vi "PH_DIM.get Boolean Status.vi"(2 "no link":bool, 3 "typeDescriptor":string, 4 "data":i8[](array[numeric]), 5 "quality":i32) -> (0 "further information":string, 1 "Status":T1 items=["no info", "off/false/out", "on/true/in", "Failure", "Alarm", "Status 1", "Status 2", "Status 3"])   [LabVIEW 2014, in "PH_Common.lvlib"]
doc: "This VI calculates the status of Boolean type DIM service. It gives out:\n\n0 (no info): no link (further information: no link)\n1 (off/false/out): link and type descriptor and quality ok, value = 0 (further information: false)\n2 (on/true/in): link and type descriptor and quality ok, value > 0 (further information: true)\n3 (Failure): link ok, type descriptor not \"S\" or \"S=1\" (further information: wrong data type) or\n link ok, type descriptor = \"S\" or \"S=1\", quality < 0 (further information: bad quality)"
uses:
  PH_StatusHandler/PH_StatusHandler.Status.ctl
  PH_Common.lvlib
  PH_StatusHandler/PH_StatusHandler.lvlib
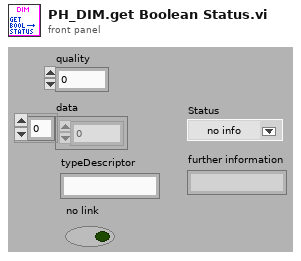
[diagram p1: front panel]
types:
  T1 = typedef "PH_StatusHandler.lvlib/PH_StatusHandler.Status.ctl" = i16
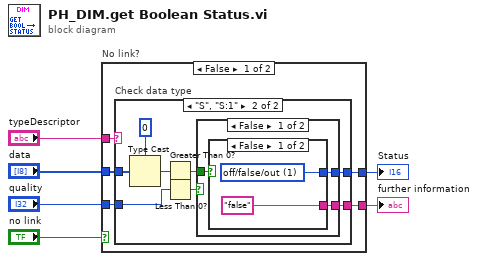
[diagram p0: block diagram]
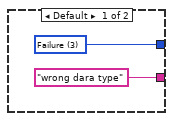
[diagram p2: hidden frame]
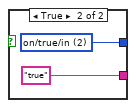
[diagram p3: hidden frame]
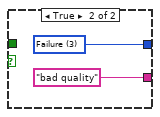
[diagram p4: hidden frame]
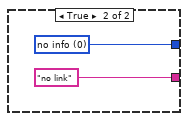
[diagram p5: hidden frame]
diagram:
  n1 = case "No link?" shown="False" "no link" {
    tunnel: [w11 w32] -> w6
    tunnel: "quality" -> [w10 _]
    tunnel: "data" -> [w9 _]
    tunnel: "typeDescriptor" -> [w8 _]
    tunnel: [w7 "no link"] -> w1
    frame False {
      n2 = case "Check data type" shown="\"S\", \"S:1\"" w8 {
        tunnel: [w13 w21] -> w11
        tunnel: w10 -> [_ w18]
        tunnel: w9 -> [_ w16]
        tunnel: ["wrong dara type" w14] -> w7
        frame Default {
          w13 = T1 3 items=["no info", "off/false/out", "on/true/in", "Failure", "Alarm", "Status 1", "Status 2", "Status 3"]
        }
        frame "S", "S:1" {
          n3 = Type Cast(type=i16 0, x=w16) -> (*(type *) &x=w15:i16)
          n4 = Greater Than 0?(x=w15) -> (x > 0?=w20:bool)
          n5 = Less Than 0?(x=w18) -> (x < 0?=w19:bool)
          n6 = case shown="False" w19 {
            tunnel: w20 -> [w24 _]
            tunnel: [w23 w30] -> w21
            tunnel: [w22 "bad quality"] -> w14
            frame False {
              n7 = case shown="False" w24 {
                tunnel: [w26 w28] -> w23
                tunnel: ["false" "true"] -> w22
                frame False {
                  w26 = T1 1 items=["no info", "off/false/out", "on/true/in", "Failure", "Alarm", "Status 1", "Status 2", "Status 3"]
                }
                frame True {
                  w28 = T1 2 items=["no info", "off/false/out", "on/true/in", "Failure", "Alarm", "Status 1", "Status 2", "Status 3"]
                }
              }
            }
            frame True {
              w30 = T1 3 items=["no info", "off/false/out", "on/true/in", "Failure", "Alarm", "Status 1", "Status 2", "Status 3"]
            }
          }
        }
      }
    }
    frame True {
      w32 = T1 0 items=["no info", "off/false/out", "on/true/in", "Failure", "Alarm", "Status 1", "Status 2", "Status 3"]
    }
  }
  "Status" <- w6
  "further information" <- w1
